vi "Self-Test.vi"(8 "error in (no error)":errorcluster, 11 "PIPXI40 Base in":refnum<class "PIPXI40 Base.lvclass">) -> (0 "error out":errorcluster, 2 "Result":variant, 3 "PIPXI40 Base out":refnum<class "PIPXI40 Base.lvclass">)   [LabVIEW 2020, in "PIPXI40.lvlib" / "PIPXI40 Base.lvclass"]
uses:
  PIPXI40 Base.lvclass
  PIPXI40 Base.lvclass/PIPXI40 Base.ctl
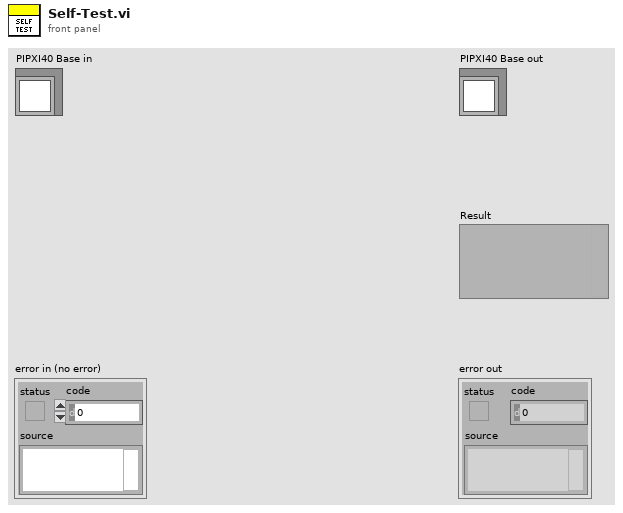
[diagram p1: front panel]
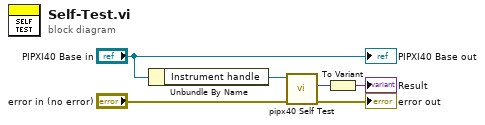
[diagram p0: block diagram]
diagram:
  n1 = Unbundle By Name("PIPXI40 Base in") -> ("Instrument handle"=w4:refnum<visa-resource-name>)
  n2 = call <instrlib>:"pipx40 Self Test.vi"("error in (no error)"="error in (no error)", "instrument handle"=w4) -> ("error out"=→"error out":errorcluster, "test result"=w1:i16)  [unwired: 6 in, 2 out]
  n3 = To Variant(anything=w1) -> (Variant=→"Result":variant)
  "PIPXI40 Base out" <- "PIPXI40 Base in"
